vi "ex_2_final.vi"() -> ()   [LabVIEW 2020]
uses:
  <vilib>/DAQmx/write.llb/DAQmx Write (Analog 1D DBL 1Chan NSamp).vi
  <vilib>/DAQmx/create/channels.llb/DAQmx Create Channel (AO-Voltage-Basic).vi
  <vilib>/DAQmx/configure/timing.llb/DAQmx Timing (Sample Clock).vi
  <vilib>/DAQmx/configure/trigger.llb/DAQmx Start Trigger (None).vi
  <vilib>/DAQmx/miscellaneous.llb/DAQmx Fill In Error Info.vi
  <vilib>/Analysis/NI_AALBase.lvlib
  <resource>/objmgr/daqmx.rc
panel:
  in  "stop":bool
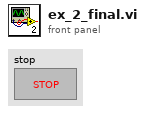
[diagram p1: front panel]
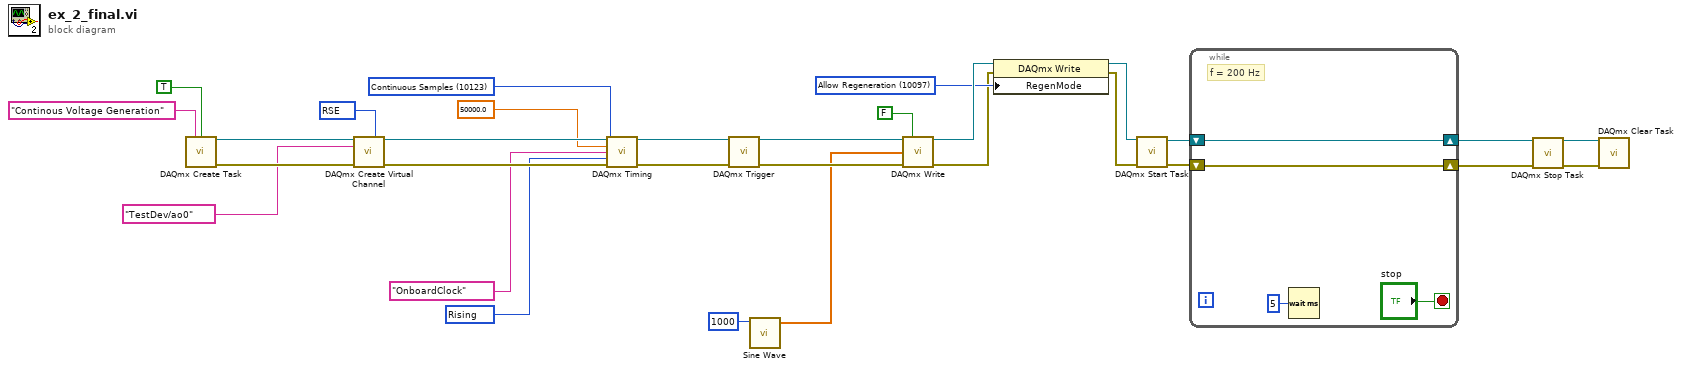
[diagram p0: block diagram]
diagram:
  w4 = 10097 items=["Allow Regeneration"=10097, "Do Not Allow Regeneration"=10158] ("RegenMode")
  w16 = 10083 items=["Default"=-1, "RSE"=10083, "NRSE"=10078, "Differential"=10106, "Pseudodifferential"=12529] ("input terminal configuration")
  w24 = 10280 items=["Rising"=10280, "Falling"=10171] ("active edge")
  w25 = 10123 items=["Finite Samples"=10178, "Continuous Samples"=10123, "Hardware Timed Single Point"=12522] ("sample mode")
  n1 = call <vilib>:"DAQmx Create Task.vi"("new task name"="Continous Voltage Generation", "auto cleanup"=TRUE) -> ("task out"=w15:refnum<k21>, "error out"=w28:errorcluster)  [unwired: 12 in]
  n2 = call-poly <vilib>:"DAQmx Create Virtual Channel.vi"("task in"=w15, "output terminal configuration"=w16, "physical channels"=tag "TestDev/ao0", "error in"=w28) -> ("task out"=w29:refnum<k21>, "error out"=w27:errorcluster)  [unwired: 10 in]
  n3 = call-poly <vilib>:"DAQmx Timing.vi"("task/channels in"=w29, "sample mode"=w25, "rate"=50000.0, "source"=tag "OnboardClock", "active edge"=w24, "error in"=w27) -> ("task out"=w20:refnum<k21>, "error out"=w19:errorcluster)  [unwired: 8 in]
  n4 = call-poly <vilib>:"DAQmx Trigger.vi"("task/channels in"=w20, "error in"=w19) -> ("task out"=w12:refnum<k21>, "error out"=w11:errorcluster)  [unwired: 12 in]
  n5 = call <vilib>:"Sine Wave.vi"("samples"=1000) -> ("sine wave"=w8:dbl[])  [unwired: 4 in, 2 out]
  n6 = call-poly <vilib>:"DAQmx Write.vi"("task/channels in"=w12, "auto start"=FALSE, "data"=w8, "error in"=w11) -> ("task out"=w6:refnum<k21>, "error out"=w3:errorcluster)  [unwired: 9 in, 1 out]
  n7 = property class="DAQmx Write"(reference=w6, error in=w3, "RegenMode"=w4) -> (reference out=w5:refnum<k21>, error out=w2:errorcluster)
  n8 = call <vilib>:"DAQmx Start Task.vi"("task/channels in"=w5, "error in"=w2) -> ("task out"=w14:refnum<k21>, "error out"=w7:errorcluster)  [unwired: 12 in]
  n9 = while {
    shift-right: [w30] -> w18
    shift-left: w14 -> [w30]
    shift-right: [w32] -> w17
    shift-left: w7 -> [w32]
    stop <- "stop" stop-if-true
    # "f = 200 Hz"
    n10 = Wait (ms)(milliseconds to wait=u32 5) -> ()  [unwired: 1 out]
  }
  n11 = call <vilib>:"DAQmx Stop Task.vi"("task/channels in"=w18) -> ("task out"=w13:refnum<k21>)  [unwired: 13 in, 1 out]
  n12 = call <vilib>:"DAQmx Clear Task.vi"("task in"=w13, "error in"=w17) -> ()  [unwired: 13 in, 1 out]
